vi "Render Draw Point.vi"(8 "error in":errorcluster, 9 "y":i32, 10 "x":i32, 11 "Renderer Pointer":u32 format="%.0x") -> (0 "error out":errorcluster, 3 "Return":i32)   [LabVIEW 2014, in "LibSDL2.lvlib"]
uses:
  LibSDL2.lvlib
  DLL/SDL2.dll
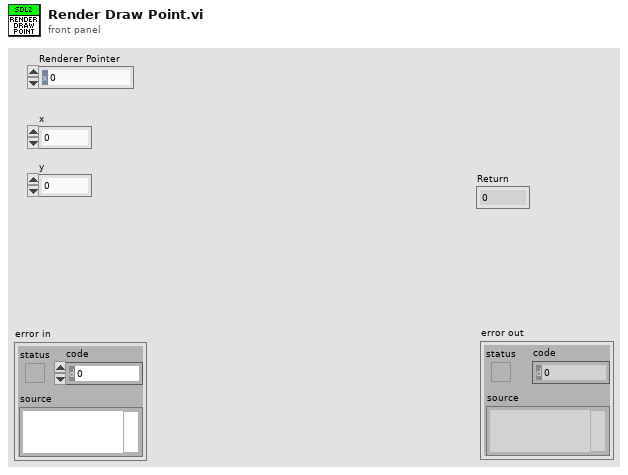
[diagram p1: front panel]
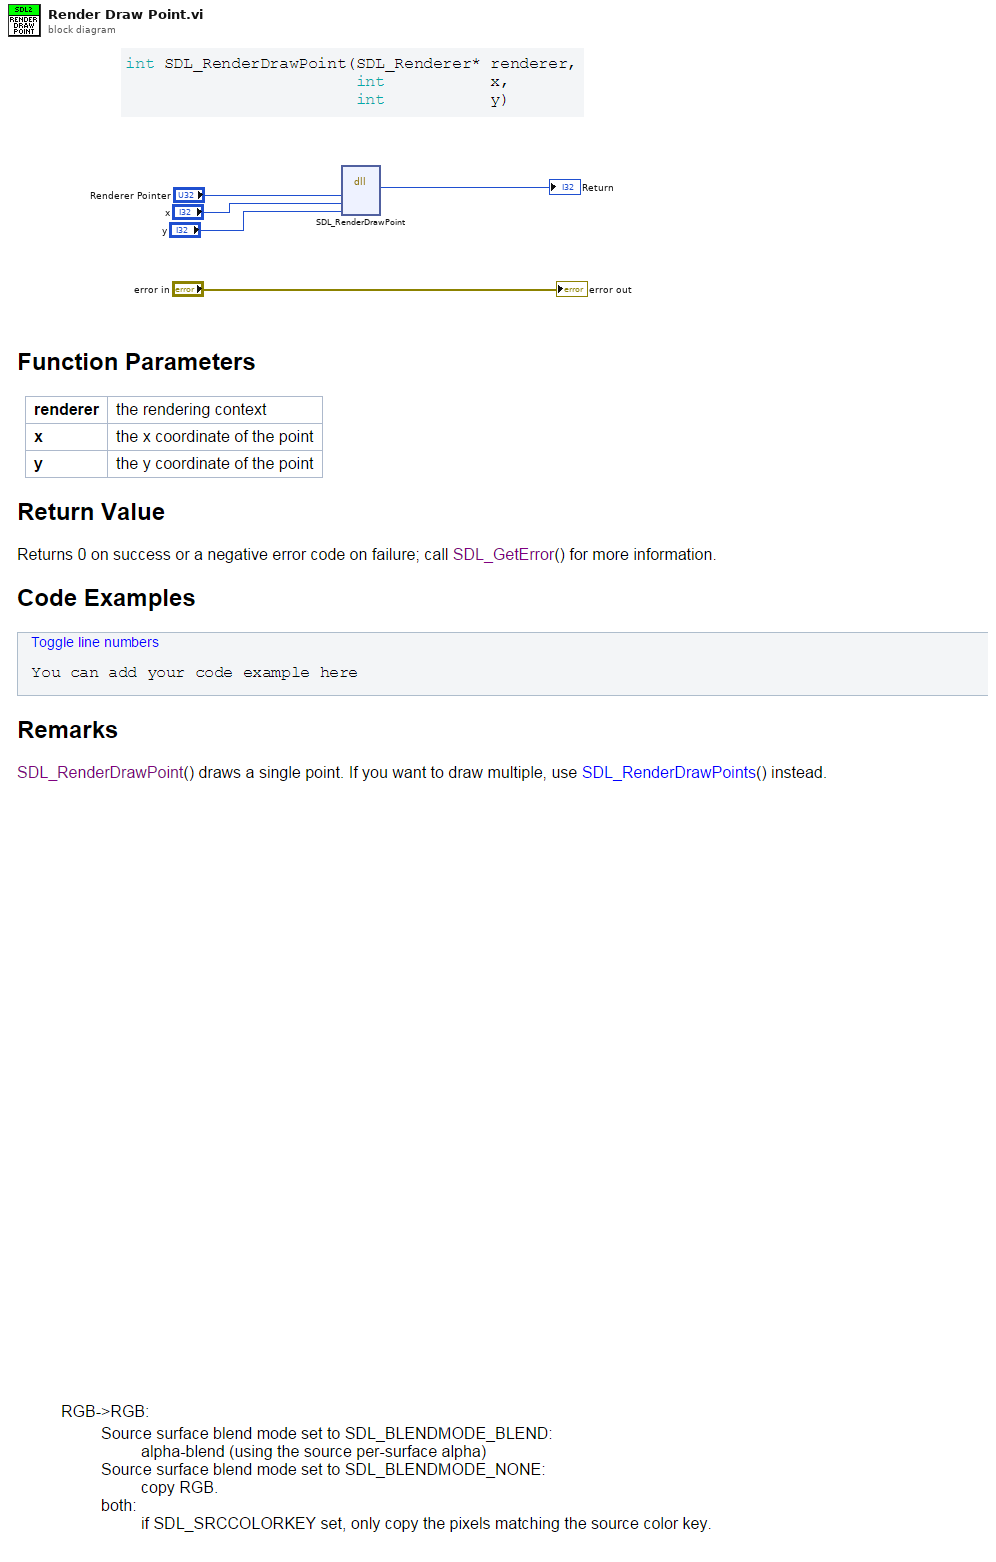
[diagram p0: block diagram]
diagram:
  n1 = dll-call lib="C:/dev/PGS/LabSDL2/Source/LibSDL2 Wrapper/DLL/SDL2.dll" fn="SDL_RenderDrawPoint"("renderer_pointer"="Renderer Pointer", "x"="x", "y"="y") -> ("return type"=→"Return":i32)  [unwired: 6 in, 2 out]
  "error out" <- "error in"
